vi "G2.vi"() -> ()   [LabVIEW 2013]
uses:
  Global test.vi
panel:
  out "Numeric":dbl
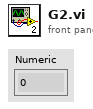
[diagram p1: front panel]
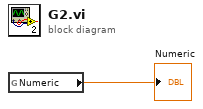
[diagram p0: block diagram]
diagram:
  n1 = global read "Global test.vi" "Numeric"() -> (→"Numeric":dbl)
